vi "GetCtrlRef.vi"(8 "error in (no error)":errorcluster, 10 "FP Control":variant, 11 "FP Controls in":refnum<class "FP Controls.lvclass">) -> (0 "error out":errorcluster, 2 "Ctrl Ref":refnum<vi>, 3 "FP Controls out":refnum<class "FP Controls.lvclass">)   [LabVIEW 2012, in "Configuration Grandmaster.lvlib" / "FP Controls.lvclass"]
uses:
  FP Controls.lvclass
  FP Controls.lvclass/FP Controls.ctl
  <vilib>/Utility/VariantDataType/VariantType.lvlib
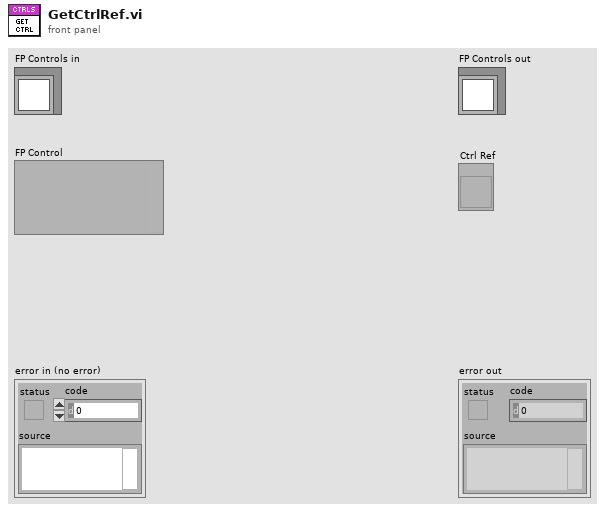
[diagram p1: front panel]
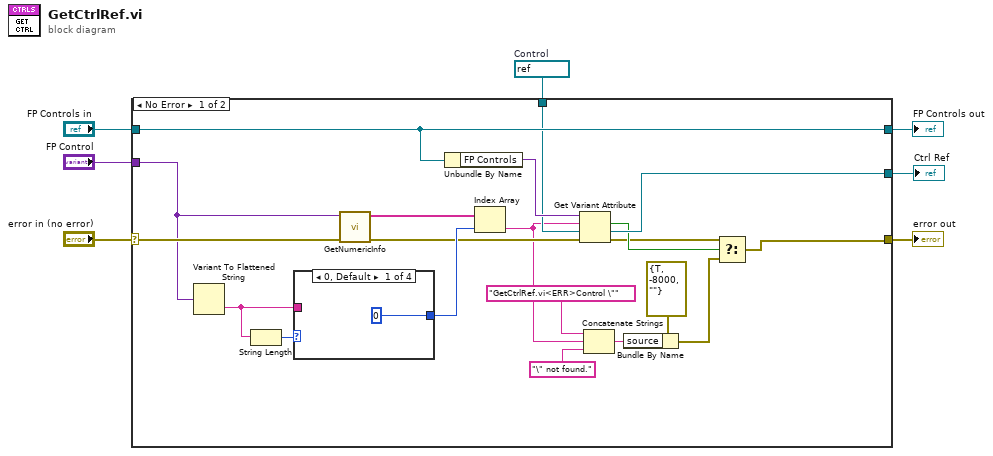
[diagram p0: block diagram]
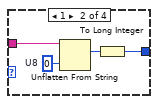
[diagram p2: hidden frame]
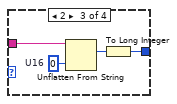
[diagram p3: hidden frame]
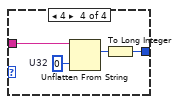
[diagram p4: hidden frame]
diagram:
  w3 = refnum<vi> refnum  # Control
  n1 = case shown="No Error" "error in (no error)" {
    selector: "error in (no error)" -> [w10 w43]
    tunnel: [w21 w43] -> w6
    tunnel: [w27 w42] -> w4
    tunnel: "FP Controls in" -> [w27 w42]
    tunnel: w3 -> [w25 w41]
    tunnel: [w24 w41] -> w2
    tunnel: "FP Control" -> [w9 _]
    frame No Error {
      n2 = Variant To Flattened String(Variant=w9) -> (data string=w13:string)  [unwired: 1 out]
      n3 = String Length(string=w13) -> (length=w12:i32)
      n4 = case shown="0, Default" w12 {
        tunnel: w13 -> [_ w32 w36 w40]
        tunnel: [0 ("U32") w29 w33 w37] -> w14
        frame 0, Default {
        }
        frame 1 {
          w31 = u8 0  # U8
          n5 = Unflatten From String(type=w31, binary string=w32) -> (value=w30:u8)  [unwired: 3 in, 2 out]
          n6 = To Long Integer(number=w30) -> (32bit integer=w29:i32)
        }
        frame 2 {
          w35 = u16 0  # U16
          n7 = Unflatten From String(type=w35, binary string=w36) -> (value=w34:u16)  [unwired: 3 in, 2 out]
          n8 = To Long Integer(number=w34) -> (32bit integer=w33:i32)
        }
        frame 4 {
          w39 = u32 0  # U32
          n9 = Unflatten From String(type=w39, binary string=w40) -> (value=w38:u32)  [unwired: 3 in, 2 out]
          n10 = To Long Integer(number=w38) -> (32bit integer=w37:i32)
        }
      }
      n11 = call <vilib>:"GetNumericInfo.vi"("error in (no error)"=w10, "Variant"=w9) -> ("error out"=w11:errorcluster, "EnumNames"=w15:string[])  [unwired: 6 in, 2 out]
      n12 = Unbundle By Name(w27) -> ("FP Controls"=w26:variant)
      n13 = Index Array(array=w15, index=w14) -> (element=w8:string)
      n14 = Get Variant Attribute(Variant=w26, name=w8, default value (empty Variant)=w25, error in=w11) -> (found=w23:bool, value=w24:refnum<vi>, error out=w22:errorcluster)  [unwired: 1 out]
      n15 = Concatenate Strings("GetCtrlRef.vi<ERR>Control \"" ("source"), w8, "\" not found." ("source")) -> (w19:string)
      n16 = Bundle By Name(cluster=errorcluster {"status"=TRUE, "code"=-8000, "source"=""} ("error out"), "source"=w19) -> (w16:errorcluster)
      n17 = Select(t=w22, s=w23, f=w16) -> (s? t:f=w21:errorcluster)
    }
    frame Error {
    }
  }
  "error out" <- w6
  "FP Controls out" <- w4
  "Ctrl Ref" <- w2
